vi "Convert AcquireParams Display.vi"(1 "ACQUIPARAMS Display":T6, 2 "ACQUIPARAMS [in]":T1 {"CFA"."CFA" items=["CFA_NONE", "CFA_VRI", "CFA_VRIV6", "CFA_BAYER", "CFA_BAYERFLIP"]; "TriggerTime"."fractions" format="%32.0f"}) -> (0 "ACQUIPARAMS [out]":T1 {"CFA"."CFA" items=["CFA_NONE", "CFA_VRI", "CFA_VRIV6", "CFA_BAYER", "CFA_BAYERFLIP"]; "TriggerTime"."fractions" format="%32.0f"})   [LabVIEW 2013, in "VRI.lvlib"]
uses:
  VRI.lvlib
  _Type Defs/PHCon ACQUIPARAMS.ctl
  _Type Defs/PhCon SyncImaging.ctl
  _Type Defs/Rect.ctl
  _Type Defs/PHCon Time64.ctl
  _Type Defs/PhInt CFA.ctl
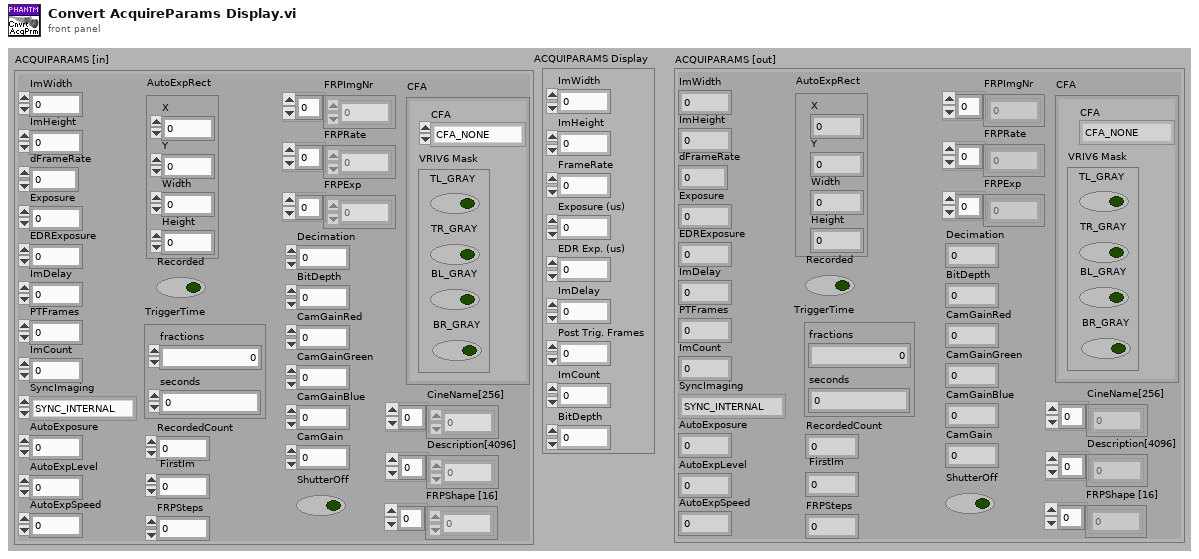
[diagram p1: front panel]
types:
  T1 = typedef "VRI.lvlib/PHCon ACQUIPARAMS.ctl" = cluster{"ImWidth":u32, "ImHeight":u32, "(deprecated)FrameRateInt":u32, "Exposure":u32, "EDRExposure":u32, "ImDelay":u32, "PTFrames":u32, "ImCount":u32, "SyncImaging":T2, "AutoExposure":u32, "AutoExpLevel":u32, "AutoExpSpeed":u32, "AutoExpRect":T3, "Recorded":bool, "TriggerTime":T4, "RecordedCount":u32, "FirstIm":i32, "FRPSteps":u32, "FRPImgNr":i32[], "FRPRate":u32[], "FRPExp":u32[], "Decimation":u32, "BitDepth":u32, "CamGainRed":u32, "CamGainGreen":u32, "CamGainBlue":u32, "CamGain":u32, "ShutterOff":bool, "CFA":T5, "CineName[256]":u8[], "Description[4096]":u8[], "FRPShape [16]":u32[], "dFrameRate":dbl}
  T2 = typedef "VRI.lvlib/PhCon SyncImaging.ctl" = enum32{"SYNC_INTERNAL", "SYNC_EXTERNAL", "SYNC_LOCKTOIRIG"}
  T3 = typedef "VRI.lvlib/Rect.ctl" = cluster{"X":i32, "Y":i32, "Width":i32, "Height":i32}
  T4 = typedef "VRI.lvlib/PHCon Time64.ctl" = cluster{"fractions":u32, "seconds":u32}
  T5 = typedef "VRI.lvlib/PhInt CFA.ctl" = cluster{"CFA":u32, "VRIV6 Mask":cluster{"TL_GRAY":bool, "TR_GRAY":bool, "BL_GRAY":bool, "BR_GRAY":bool}}
  T6 = cluster{"ImWidth":u32, "ImHeight":u32, "FrameRate":u32, "Exposure (us)":u32, "EDR Exp. (us)":u32, "ImDelay":u32, "Post Trig. Frames":u32, "ImCount":u32, "BitDepth":u32}
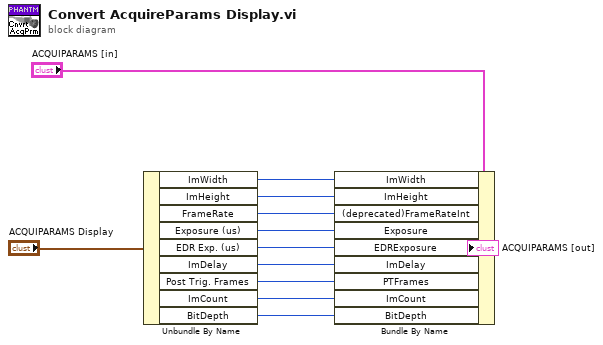
[diagram p0: block diagram]
diagram:
  n1 = Unbundle By Name("ACQUIPARAMS Display") -> ("ImWidth"=w10:u32, "ImHeight"=w9:u32, "FrameRate"=w8:u32, "Exposure (us)"=w2:u32, "EDR Exp. (us)"=w1:u32, "ImDelay"=w7:u32, "Post Trig. Frames"=w6:u32, "ImCount"=w5:u32, "BitDepth"=w4:u32)
  n2 = Bundle By Name(cluster="ACQUIPARAMS [in]", "ImWidth"=w10, "ImHeight"=w9, "(deprecated)FrameRateInt"=w8, "Exposure"=w2, "EDRExposure"=w1, "ImDelay"=w7, "PTFrames"=w6, "ImCount"=w5, "BitDepth"=w4) -> (→"ACQUIPARAMS [out]":T1)
